vi "SMU_Meas and Calculate Resitance_No Publish_Source and Sink_w updated Par Calc.vi"(7 "Current  Level":dbl=0.01, 8 "error in (no error)":errorcluster, 10 "Pins":string[](array[string]), 11 "Semiconductor Module Context":T1) -> (0 "error Out":errorcluster, 1 "Parallel_Resitance":dbl[](array[numeric]), 2 "R Array":dbl[](array[numeric]), 3 "Semiconductor Module Context Out":T1)   [LabVIEW 2013]
uses:
  <vilib>/NI_TestStand_SemiconductorModule/NI_TestStand_Semiconductor_Module.lvlibp/PinMap/General/SemiconductorModuleContext.ctl
  <vilib>/NI_TestStand_SemiconductorModule/NI_TestStand_Semiconductor_Module.lvlibp/PinMap/DC Power/PinsToNIDCPowerSessions.vi
  <vilib>/NI_TestStand_SemiconductorModule/NI_TestStand_Semiconductor_Module.lvlibp
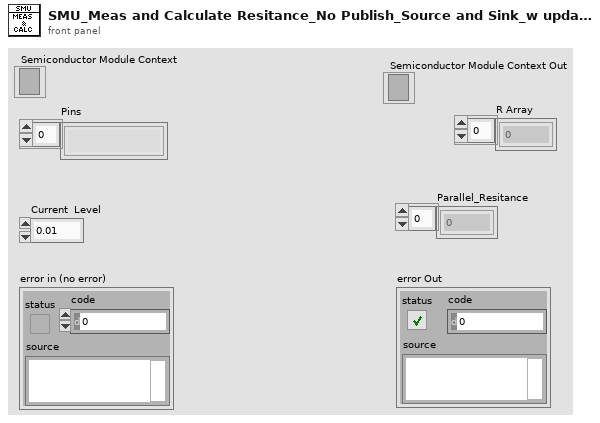
[diagram p1: front panel]
types:
  T1 = typedef "NI_TestStand_Semiconductor_Module.lvlibp/SemiconductorModuleContext.ctl" = refnum<k7>
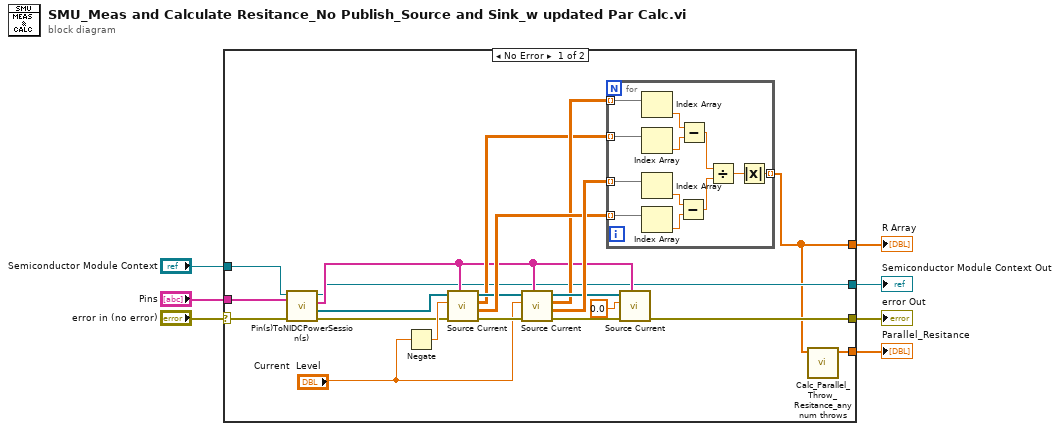
[diagram p0: block diagram]
diagram:
  n1 = case shown="No Error" "error in (no error)" {
    selector: "error in (no error)" -> [w28 w42]
    tunnel: "Semiconductor Module Context" -> [w18 w41]
    tunnel: "Pins" -> [w19 _]
    tunnel: [w11 w42] -> w4
    tunnel: [w10 w41] -> w3
    tunnel: [w9 _] -> w2
    tunnel: [w8 _] -> w1
    frame No Error {
      n2 = call-poly <vilib>:"Pin(s)ToNIDCPowerSession(s).vi"("error in (no error)"=w28, "Pins"=w19, "Semiconductor Module Context"=w18) -> ("error out"=w14:errorcluster, "Instrument Sessions"=w13:refnum<k15>[], "Channel Lists"=w15:string[], "Semiconductor Module Context Out"=w10:T1)  [unwired: 4 in, 1 out]
      n3 = Negate(x="Current  Level") -> (-x=w24:dbl)
      n4 = call "Source Current.vi"("Channel Lists"=w15, "error in (no error)"=w14, "current level"=w24, "Instrument Sessions In"=w13) -> ("error out"=w22:errorcluster, "current measurements"=w26:dbl[][], "voltage measurements"=w20:dbl[][], "Instrument Sessions Out"=w21:refnum<k15>[])  [unwired: 4 in]
      n5 = call "Source Current.vi"("Channel Lists"=w15, "error in (no error)"=w22, "current level"="Current  Level", "Instrument Sessions In"=w21) -> ("error out"=w17:errorcluster, "current measurements"=w27:dbl[][], "voltage measurements"=w23:dbl[][], "Instrument Sessions Out"=w25:refnum<k15>[])  [unwired: 4 in]
      n6 = for {
        tunnel: w23 -> [w32] mode=indexing
        tunnel: w27 -> [w40] mode=indexing
        tunnel: [w38] -> w9 mode=indexing
        tunnel: w26 -> [w36] mode=indexing
        tunnel: w20 -> [w29] mode=indexing
        n7 = Index Array(array=w32) -> (element=w31:dbl)  [unwired: 1 in]
        n8 = Index Array(array=w29) -> (element=w30:dbl)  [unwired: 1 in]
        n9 = Index Array(array=w40) -> (element=w33:dbl)  [unwired: 1 in]
        n10 = Index Array(array=w36) -> (element=w35:dbl)  [unwired: 1 in]
        n11 = Subtract(x=w33, y=w35) -> (x-y=w34:dbl)
        n12 = Subtract(x=w31, y=w30) -> (x-y=w37:dbl)
        n13 = Divide(x=w37, y=w34) -> (x/y=w39:dbl)
        n14 = Absolute Value(x=w39) -> (abs(x)=w38:dbl)
      }
      n15 = call "Source Current.vi"("Channel Lists"=w15, "error in (no error)"=w17, "current level"=0.0, "Instrument Sessions In"=w25) -> ("error out"=w11:errorcluster)  [unwired: 4 in, 3 out]
      n16 = call "Calc_Parallel_Throw_Resitance_any num throws.vi"("Resitance_Per Site"=w9) -> ("Parallel_Resitance"=w8:dbl[])  [unwired: 10 in]
    }
    frame Error {
    }
  }
  "error Out" <- w4
  "Semiconductor Module Context Out" <- w3
  "R Array" <- w2
  "Parallel_Resitance" <- w1
